vi "Example_ImageToArray.vi"() -> ()   [LabVIEW 2020, in "OpenLvVision_Image.lvlib"]
uses:
  OpenLvVision_Image.lvlib
  Management/TypeDef/ImageType.ctl
  DataAccess/TypeDef/RectangleI32.ctl
  DataAccess/ImageToArray/ImageMonoU8ToArray.vi
  Management/Management.lvlib
  File/File.lvlib
  DataAccess/DataAccess.lvlib
panel:
  in  "Image Path":path
  out "Pixel":u8[][](array[numeric])
  out "Image":T1(plugin-control)
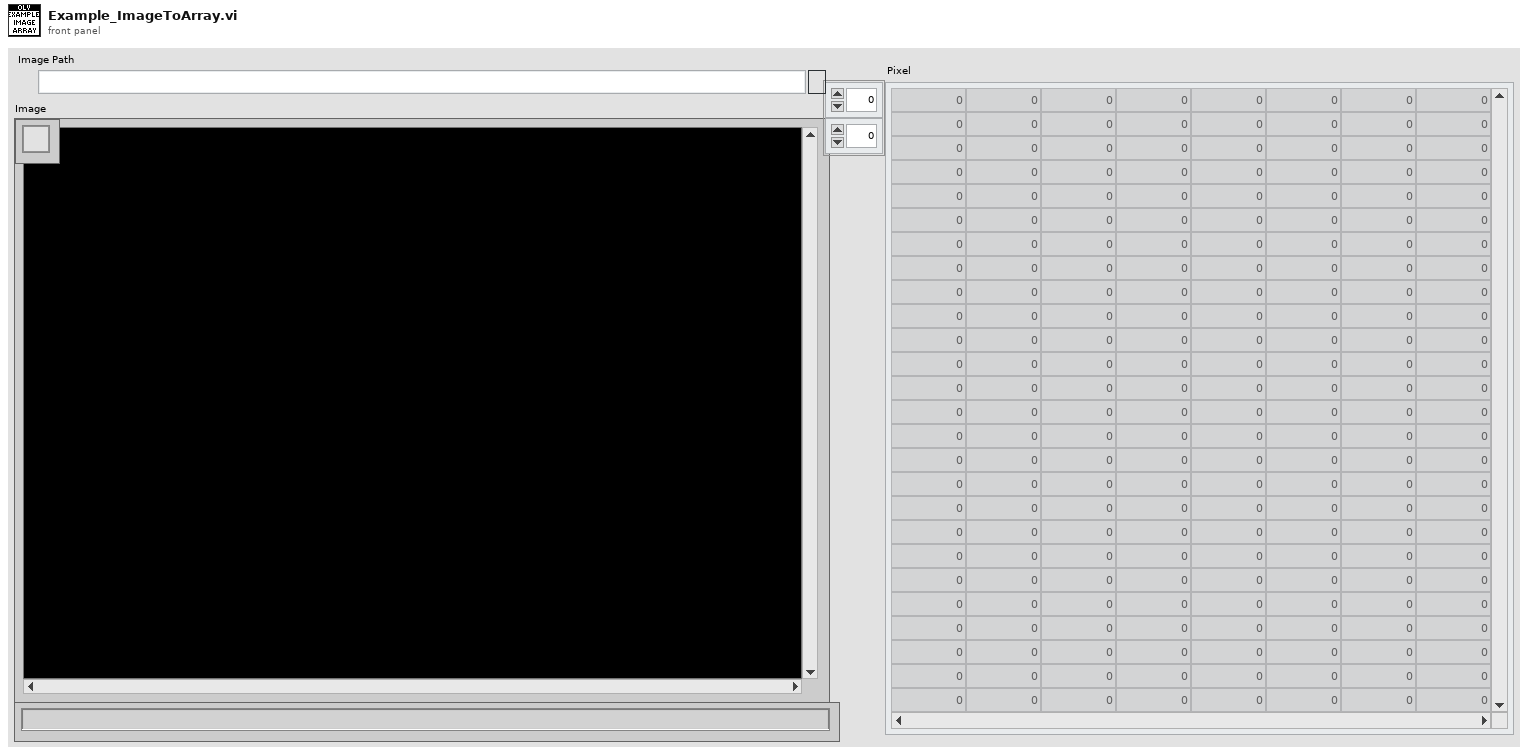
[diagram p1: front panel]
types:
  T1 = typedef "IMAQ Image.ctl" = refnum<image>
  T2 = typedef "OpenLvVision_Image.lvlib/Management.lvlib/ImageType.ctl" = enum16{"Mono U8", "Mono U16", "Mono I16", "Mono SGL", "Color U32", "Color U64", "Complex CSG"}
  T3 = typedef "OpenLvVision_Image.lvlib/Management.lvlib/Image.ctl" = refnum<image>
  T4 = typedef "OpenLvVision_Image.lvlib/DataAccess.lvlib/RectangleI32.ctl" = cluster{"Left":i32, "Top":i32, "Right":i32, "Bottom":i32}
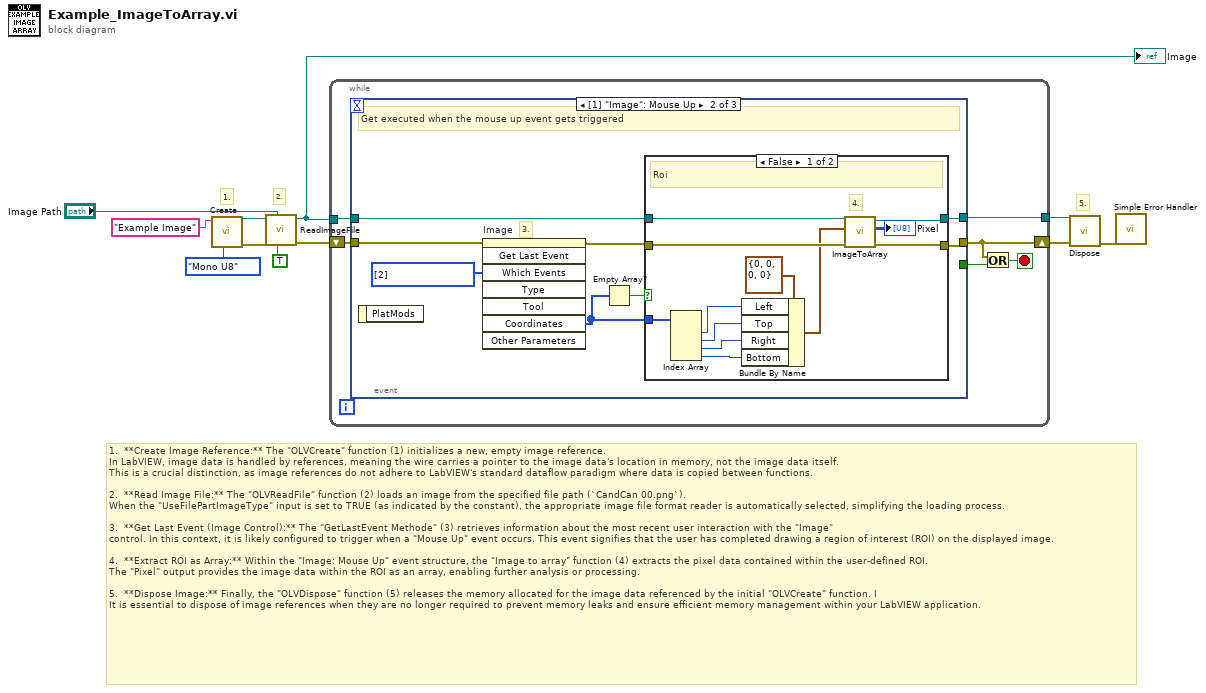
[diagram p0: block diagram]
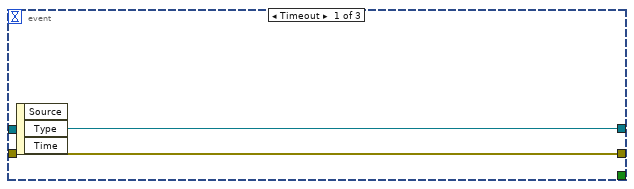
[diagram p2: hidden frame]
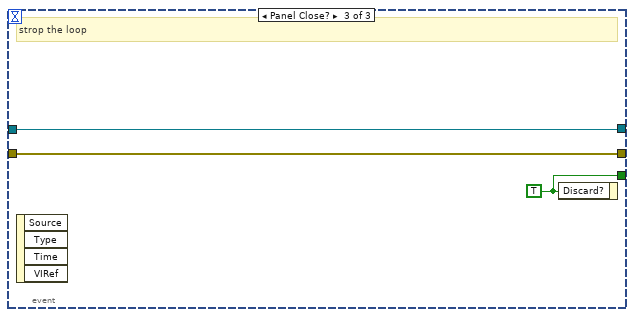
[diagram p4: hidden frame]
diagram:
  # "1.  **Create Image Reference:** The \"OLVCreate\" function (1) initializes a new, empty image reference. \nIn LabVIEW, image data is handled by references, meaning the wire carries a pointer to the image data's location in memory, not the image data itself. \nThis is a crucial distinction, as image references do not adhere to LabVIEW's standard dataflow paradigm where data is copied between functions.\n\n2.  **Read Image File:** The \"OLVReadFile\" function (2) loads an image from the specified file path (`CandCan 00.png`). \nWhen the \"UseFilePartImageType\" input is set to TRUE (as indicated by the constant), the appropriate image file format reader is automatically selected, simplifying the loading process.\n\n3.  **Get Last Event (Image Control):** The \"GetLastEvent Methode\" (3) retrieves information about the most recent user interaction with the \"Image\" \ncontrol. In this context, it is likely configured to trigger when a \"Mouse Up\" event occurs. This event signifies that the user has completed drawing a region of interest (ROI) on the displayed image.\n\n4.  **Extract ROI as Array:** Within the \"Image: Mouse Up\" event structure, the \"Image to array\" function (4) extracts the pixel data contained within the user-defined ROI. \nThe \"Pixel\" output provides the image data within the ROI as an array, enabling further analysis or processing.\n\n5.  **Dispose Image:** Finally, the \"OLVDispose\" function (5) releases the memory allocated for the image data referenced by the initial \"OLVCreate\" function. I\nIt is essential to dispose of image references when they are no longer required to prevent memory leaks and ensure efficient memory management within your LabVIEW application."
  # "5."
  # "2."
  # "1."
  n1 = call "Create.vi"("Image Type"=ImageType."Mono U8", "Image Name"="Example Image") -> ("error out"=w8:errorcluster, "Image Reference Out"=w7:T3)  [unwired: 8 in]
  n2 = call "ReadImageFile.vi"("Use File Path Image Type"=TRUE, "File Path"="Image Path", "error in"=w8, "Image Reference In"=w7) -> ("error out"=w5:errorcluster, "Image Reference Out"=w6:T3)  [unwired: 3 in, 3 out]
  "Image" <- w6
  n3 = while {
    tunnel: w6 -> [w17]
    shift-right: [w14] -> w4
    shift-left: w5 -> [w16]
    tunnel: [w15] -> w2
    stop <- w13 stop-if-true
    n4 = event shown="[1] \"Image\": Mouse Up" {
      selector: _ -> [_ _ _]
      dyn-events: _ -> [_ _ _]
      timeout: _ -> [_ _ _]
      tunnel: w17 -> [w19 w25 w44]
      tunnel: w16 -> [w18 w27 w43]
      tunnel: [w18 w22 w43] -> w14
      tunnel: [w19 w23 w44] -> w15
      tunnel: [_ _ w42] -> w12
      event Timeout {
        n5 = event-data() -> ()  [unwired: 1 in, 3 out]
      }
      event "Image": Mouse Up {
        w26 = i32[] [2] items=["No Event"=0, "Click Event"=1, "Draw Event"=2, "Size Event"=4, "Scroll Event"=5, "Double Click Event"=8] ("Which Events")
        # "3."
        # "Get executed when the mouse up event gets triggered"
        n6 = event-data() -> ()  [unwired: 1 in, 1 out]
        n7 = invoke on="Image" class="ImageControl" method="Get Last Event"(error in=w27, "Which Events"=w26) -> (error out=w24:errorcluster, "Coordinates"=w20:i32[])  [unwired: 6 in, 6 out]
        n8 = Empty Array?(array=w20) -> (empty?=w21:bool)
        n9 = case shown="False" w21 {
          tunnel: w25 -> [w37 w41]
          tunnel: w24 -> [w36 w40]
          tunnel: [w38 w41] -> w23
          tunnel: [w39 w40] -> w22
          tunnel: w20 -> [w33 _]
          frame False {
            # "4."
            # "Roi"
            n10 = Index Array(array=w33) -> (element #1=w32:i32, element #2=w31:i32, element #3=w30:i32, element #4=w29:i32)  [unwired: 4 in]
            n11 = Bundle By Name(cluster=T4 {"Left"=0, "Top"=0, "Right"=0, "Bottom"=0} ("Optional Rectangle"), "Left"=w32, "Top"=w31, "Right"=w30, "Bottom"=w29) -> (w34:T4)
            n12 = call-poly "ImageToArray.vi"("error in"=w36, "Optional Rectangle"=w34, "Image Reference In"=w37) -> ("error out"=w39:errorcluster, "Pixel"=→"Pixel":u8[][], "Image Reference Out"=w38:T3)  [unwired: 6 in]
          }
          frame True {
            # "Roi empty"
          }
        }
      }
      event Panel Close? {
        w42 = TRUE
        # "strop the loop"
        n13 = event-data() -> ()  [unwired: 1 in, 4 out]
        n14 = event-data("Discard?"=w42) -> ()  [unwired: 1 in, 1 out]
      }
    }
    n15 = Or(x=w14, y=w12) -> (x .or. y?=w13:bool)
  }
  n16 = call "Dispose.vi"("error in"=w4, "Image Reference In"=w2) -> ("error out"=w3:errorcluster)  [unwired: 9 in]
  n17 = call <vilib>:"Simple Error Handler.vi"("error in (no error)"=w3) -> ()  [unwired: 4 in, 5 out]
